vi "DDS Startup.vi"(8 "error in (no error)":errorcluster, 11 "DDS.lvclass (in)":refnum<class "DDS.lvclass">) -> (0 "error out":errorcluster, 3 "DDS.lvclass":refnum<class "DDS.lvclass">)   [LabVIEW 2013, in "DDS.lvclass"]
uses:
  cesium_controller/DDS/DDS.lvclass
  cesium_controller/DDS/DDS.lvclass/DDS.ctl
  cesium_controller/Experiment/Globals.vi
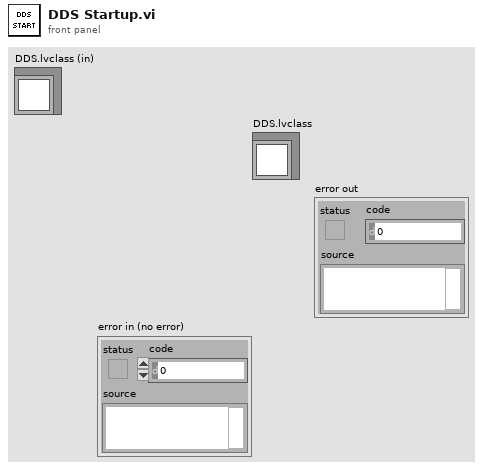
[diagram p1: front panel]
types:
  T1 = typedef "Array_of_DDS_Boxes.ctl" = T2[]
  T2 = typedef "DDS_box_cluster.ctl" = cluster{"DDS box device reference":T3, "Array of DDS Channels (4)":T5, "Enable":bool, "Description":string}
  T3 = typedef "DDS_box_device_reference.ctl" = cluster{"NI USB-8451 device reference":T4, "DIO port":u8, "Serial Clock Rate [kHz]":u16}
  T4 = typedef "ni845xControl.ctl" = refnum<k21>
  T5 = typedef "DDS.lvclass/array_of_DDS_channels.ctl" = T6[]
  T6 = typedef "DDS.lvclass/DDS_channel.ctl" = cluster{"Power":bool, "Channel Parameters":cluster{"Ref Clock Rate [kHz]":dbl, "Full Scale Output\nPower [dBm]":dbl}, "RAM Enable":bool, "RAM Dest Type":u8, "RAM Default":cluster{"Frequency [MHz]":dbl, "Amplitude [dBm]":dbl, "Phase Offset [rad]":dbl}, "Array of DDS Profiles (8)":T7, "Description":string}
  T7 = typedef "DDS.lvclass/array_of_DDS_profiles.ctl" = T8[]
  T8 = typedef "DDS_profile.ctl" = cluster{"Single Tone":cluster{"Frequency [MHz]":dbl, "Amplitude [dBm]":dbl, "Phase Offset [rad]":dbl}, "RAM Mode ":T9, "Zero-crossing":bool, "No Dwell High":bool, "Function/Static":bool, "RAM Function Settings":string[], "RAM Static Array":dbl[], "Description":string}
  T9 = typedef "DDS RAM mode.ctl" = enum16{"Direct Switch", "Ramp Up", "Bidirectional Ramp", "Continuous Bidirectional Ramp", "Continuous Recirculate", "Direct Switch 2", "Direct Switch 3", "Direct Switch 4"}
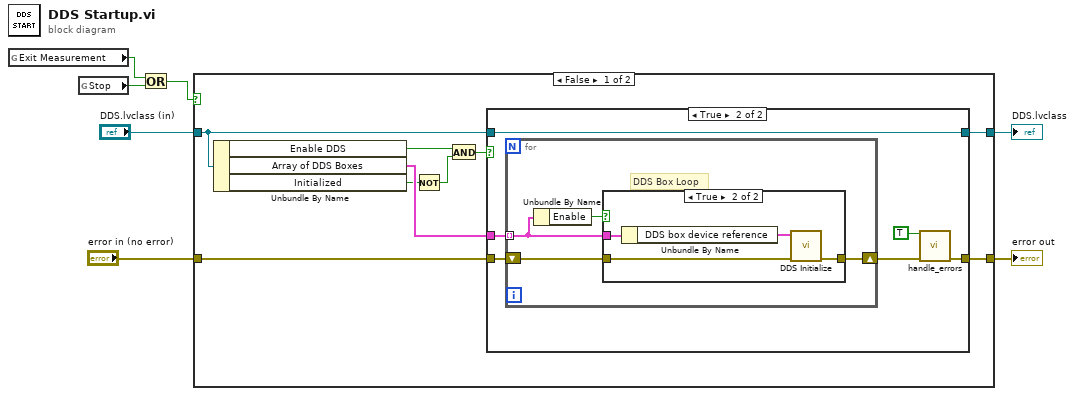
[diagram p0: block diagram]
diagram:
  n1 = global read "Globals.vi" "Exit Measurement"() -> (w4:bool)
  n2 = global read "Globals.vi" "Stop"() -> (w3:bool)
  n3 = Or(x=w4, y=w3) -> (x .or. y?=w2:bool)
  n4 = case shown="False" w2 {
    tunnel: "error in (no error)" -> [w16 w35]
    tunnel: [w14 w35] -> w6
    tunnel: "DDS.lvclass (in)" -> [w13 w34]
    tunnel: [w12 w34] -> w1
    frame False {
      n5 = Unbundle By Name(w13) -> ("Enable DDS"=w11:bool, "Array of DDS Boxes"=w15:T1, "Initialized"=w9:bool)
      n6 = Not(x=w9) -> (.not. x?=w10:bool)
      n7 = And(x=w11, y=w10) -> (x .and. y?=w8:bool)
      n8 = case shown="True" w8 {
        tunnel: [w18 w21] -> w14
        tunnel: w16 -> [w18 w24]
        tunnel: w15 -> [_ w23]
        tunnel: w13 -> [w17 w20]
        tunnel: [w17 w20] -> w12
        frame False {
        }
        frame True {
          n9 = for {
            shift-right: [w25] -> w19
            shift-left: w24 -> [w26]
            tunnel: w23 -> [w27] mode=indexing
            # "DDS Box Loop"
            n10 = Unbundle By Name(w27) -> ("Enable"=w28:bool)
            n11 = case shown="True" w28 {
              tunnel: w27 -> [_ w33]
              tunnel: w26 -> [w29 w32]
              tunnel: [w29 w30] -> w25
              frame False {
              }
              frame True {
                n12 = Unbundle By Name(w33) -> ("DDS box device reference"=w31:T3)
                n13 = call "DDS Initialize.vi"("error in (no error)"=w32, "DDS ref in"=w31) -> ("error out"=w30:errorcluster)  [unwired: 8 in, 1 out]
              }
            }
          }
          n14 = call "handle_errors.vi"("Exit Operation"=TRUE ("Exit Measurement"), "error in (no error)"=w19) -> ("error out"=w21:errorcluster)  [unwired: 13 in]
        }
      }
    }
    frame True {
    }
  }
  "error out" <- w6
  "DDS.lvclass" <- w1
